vi "Drive Back.vi"(4 "Time":dbl=1.0, 6 "Speed":dbl=1.0, 11 "error in":errorcluster) -> (3 "error out":errorcluster)   [LabVIEW 2015]
uses:
  References/Refnums.vi
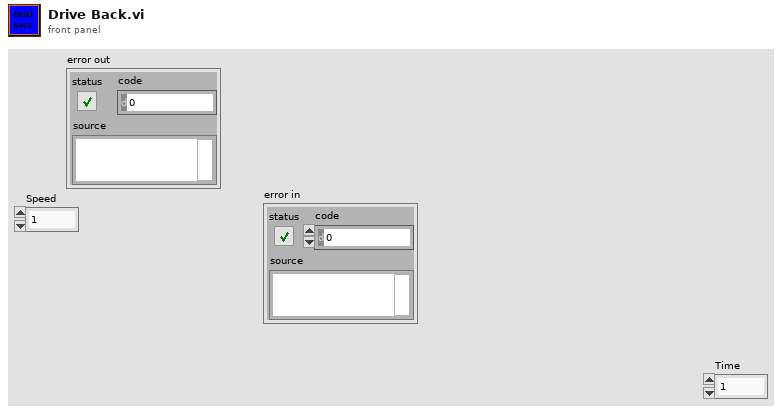
[diagram p1: front panel]
types:
  T1 = typedef "WPI_MotorControlDeviceRef.ctl" = cluster{"DeviceStatus":errorcluster, "Type":T2, "PWM":cluster{"PWM Channel":T3, "DeadBand":T4}, "CAN":cluster{"Device Number":u8, "Control Mode":T5, "Semaphore":T6, "Max Vout":dbl, "TalonSRX Control Mode":T7}, "Invert":bool}
  T2 = typedef "WPI_MotorControlType.ctl" = enum16{"PWM", "CAN", "CANTalonSRX"}
  T3 = typedef "FPGA_DIOPWMChannel.ctl" = enum8{"PWM 0", "PWM 1", "PWM 2", "PWM 3", "PWM 4", "PWM 5", "PWM 6", "PWM 7", "PWM 8", "PWM 9", "PWM MXP 0", "PWM MXP 1", "PWM MXP 2", "PWM MXP 3", "PWM MXP 4", "PWM MXP 5", "PWM MXP 6", "PWM MXP 7", "PWM MXP 8", "PWM MXP 9", "Invalid"}
  T4 = typedef "WPI_PWMDeadband.ctl" = cluster{"Name":string, "maxPositivePwm":i32, "minPositivePwm":i32, "centerPwm":i32, "maxNegativePwm":i32, "minNegativePwm":i32, "angularRange":u16}
  T5 = typedef "WPI_CANJaguar_ControlMode.ctl" = enum8{"Percent VBus", "Current", "Speed", "Position", "Voltage"}
  T6 = typedef "Semaphore RefNum" = refnum<k1>
  T7 = typedef "WPI_CANTalonSRX_APIControlMode.ctl" = enum8{"Percent VBus", "Speed", "Position", "Slave", "Unchanged / Invalid", "Voltage Compensation", "Current", "Motion Profile"}
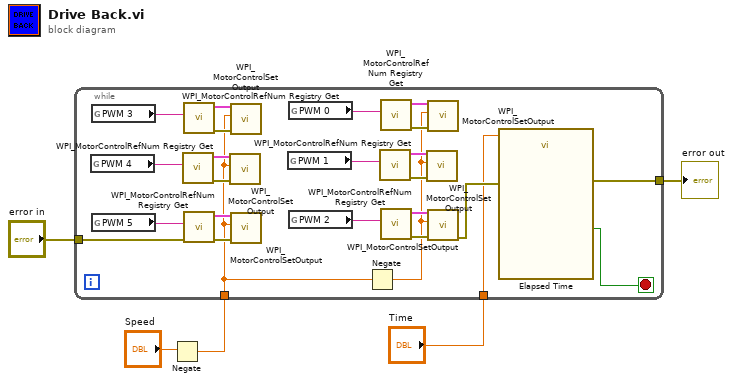
[diagram p0: block diagram]
diagram:
  n1 = Negate(x="Speed") -> (-x=w1:dbl)
  n2 = while {
    tunnel: [w10] -> w5
    tunnel: "error in" -> [w9]
    tunnel: "Time" -> [w7]
    tunnel: w1 -> [w6]
    stop <- w12 stop-if-true
    n3 = global read "Refnums.vi" "PWM 4"() -> (w16:string)
    n4 = global read "Refnums.vi" "PWM 3"() -> (w15:string)
    n5 = global read "Refnums.vi" "PWM 5"() -> (w21:string)
    n6 = call <vilib>:"WPI_MotorControlRefNum Registry Get.vi"("refnum name"=w16) -> ("error out"=w18:errorcluster, "MotorControlDevRef"=w17:T1)  [unwired: 9 in]
    n7 = call <vilib>:"WPI_MotorControlRefNum Registry Get.vi"("refnum name"=w15) -> ("error out"=w13:errorcluster, "MotorControlDevRef"=w14:T1)  [unwired: 9 in]
    n8 = call <vilib>:"WPI_MotorControlRefNum Registry Get.vi"("error in (no error)"=w9, "refnum name"=w21) -> ("error out"=w19:errorcluster, "MotorControlDevRef"=w20:T1)  [unwired: 8 in]
    n9 = call <vilib>:"WPI_MotorControlSetOutput.vi"("error in (no error)"=w18, "Output"=w6, "MotorControlDevRef"=w17) -> ()  [unwired: 6 in, 3 out]
    n10 = call <vilib>:"WPI_MotorControlSetOutput.vi"("error in (no error)"=w13, "Output"=w6, "MotorControlDevRef"=w14) -> ()  [unwired: 6 in, 3 out]
    n11 = call <vilib>:"WPI_MotorControlSetOutput.vi"("error in (no error)"=w19, "Output"=w6, "MotorControlDevRef"=w20) -> ()  [unwired: 6 in, 3 out]
    n12 = global read "Refnums.vi" "PWM 1"() -> (w27:string)
    n13 = global read "Refnums.vi" "PWM 0"() -> (w28:string)
    n14 = global read "Refnums.vi" "PWM 2"() -> (w22:string)
    n15 = Negate(x=w6) -> (-x=w8:dbl)
    n16 = call <vilib>:"WPI_MotorControlRefNum Registry Get.vi"("refnum name"=w27) -> ("error out"=w25:errorcluster, "MotorControlDevRef"=w26:T1)  [unwired: 9 in]
    n17 = call <vilib>:"WPI_MotorControlRefNum Registry Get.vi"("refnum name"=w28) -> ("error out"=w30:errorcluster, "MotorControlDevRef"=w29:T1)  [unwired: 9 in]
    n18 = call <vilib>:"WPI_MotorControlRefNum Registry Get.vi"("refnum name"=w22) -> ("error out"=w24:errorcluster, "MotorControlDevRef"=w23:T1)  [unwired: 9 in]
    n19 = call <vilib>:"WPI_MotorControlSetOutput.vi"("error in (no error)"=w25, "Output"=w8, "MotorControlDevRef"=w26) -> ()  [unwired: 6 in, 3 out]
    n20 = call <vilib>:"WPI_MotorControlSetOutput.vi"("error in (no error)"=w30, "Output"=w8, "MotorControlDevRef"=w29) -> ()  [unwired: 6 in, 3 out]
    n21 = call <vilib>:"WPI_MotorControlSetOutput.vi"("error in (no error)"=w24, "Output"=w8, "MotorControlDevRef"=w23) -> ("error out"=w11:errorcluster)  [unwired: 6 in, 2 out]
    n22 = call "Elapsed Time"("Time Target (s)"=w7, "error in (no error)"=w11) -> ("Time has Elapsed"=w12:bool, "error out"=w10:errorcluster)  [unwired: 10 in, 6 out]
  }
  "error out" <- w5
